vi "Get XNET Signal Names.vi"(6 "Add Info?":bool, 7 "Parent Ref in":T1 format="%.0x", 8 "error in":errorcluster, 9 "Tree In":refnum<vi>, 10 "Parent":string, 11 "Frms":refnum<k21>[](array[refnum])) -> (0 "error out":errorcluster, 1 "Tree Out":refnum<vi>, 3 "XNET Signal Names":refnum<k21>[](array[refnum]))   [LabVIEW 2023, in "J1939 Addon System Explorer.lvlib"]
uses:
  J1939 Addon System Explorer.lvlib
  <vilib>/NI VeriStand/Custom Device API/Custom Device Item Ref.ctl
  <vilib>/NI VeriStand/Custom Device API/Custom Device Channel.ctl
  <vilib>/NI VeriStand/Custom Device API/Custom Device Channel Type.ctl
  Addon Shared/Types/SPN Properties.ctl
  Addon Shared/SubVIs/Constants.vi
  <vilib>/NI VeriStand/Custom Device Tools/Custom Device Utility Library/NI VeriStand - Search for Item by Name.vi
  <vilib>/NI VeriStand/Custom Device API/Set Item Property (U32).vi
  <resource>/objmgr/xnet.rc
  <vilib>/NI VeriStand/Custom Device API/Custom Device API.lvlib
  Addon Shared/J1939 Addon Shared.lvlib
  <vilib>/NI VeriStand/Custom Device Tools/Custom Device Utility Library/Custom Device Utility Library.lvlib
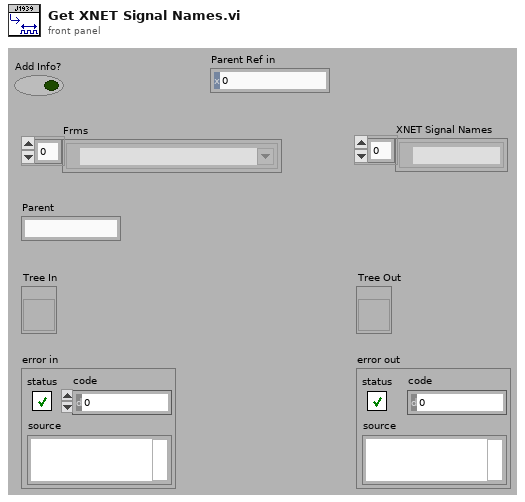
[diagram p1: front panel]
types:
  T1 = typedef "Custom Device API.lvlib/Custom Device Item Ref.ctl" = u64
  T2 = typedef "Custom Device API.lvlib/Custom Device Channel.ctl" = cluster{"Type":T3, "Units":string, "Default Value":dbl, "Faultable":bool, "Scalable":bool}
  T3 = typedef "Custom Device API.lvlib/Custom Device Channel Type.ctl" = enum16{"Input", "Output"}
  T4 = typedef "J1939 Addon Shared.lvlib/SPN Properties.ctl" = cluster{"Bytes":u32, "ScaleFac":dbl, "ScaleOff":dbl}
  T5 = typedef "Custom Device API.lvlib/Custom Device Item Info.ctl" = cluster{"Name":string, "Is Channel":bool, "GUID":string, "Is Waveform":bool}
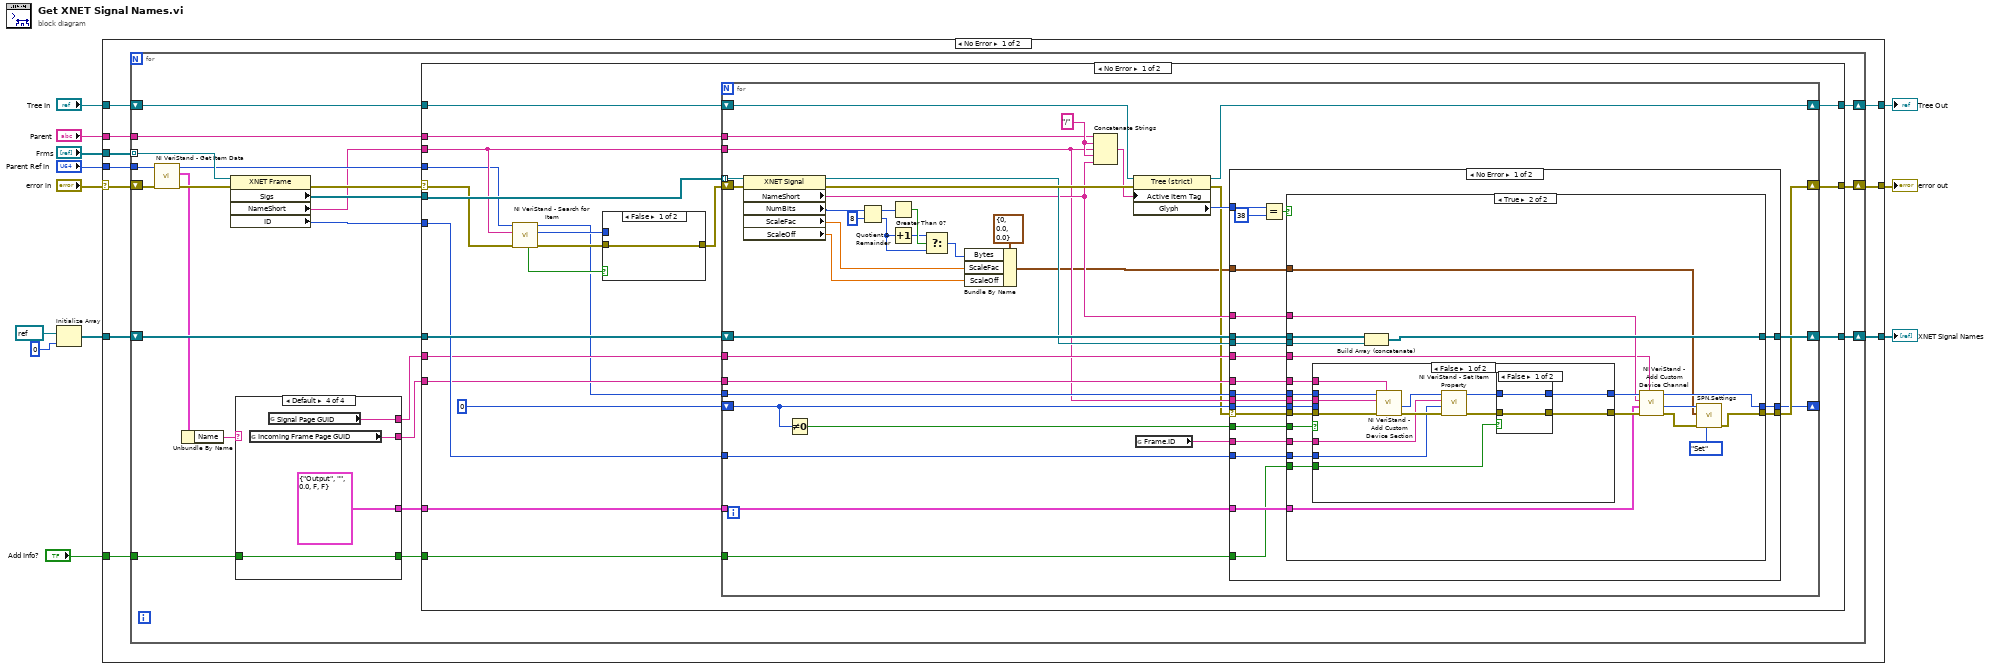
[diagram p0: block diagram]
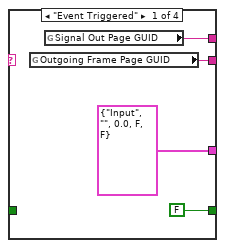
[diagram p2: hidden frame]
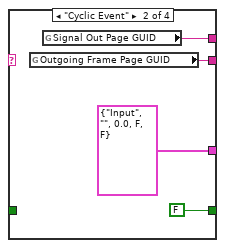
[diagram p3: hidden frame]
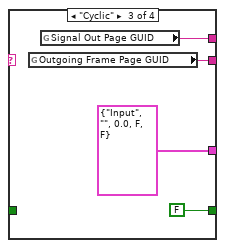
[diagram p4: hidden frame]
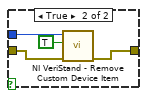
[diagram p5: hidden frame]
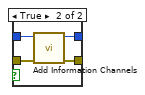
[diagram p7: hidden frame]
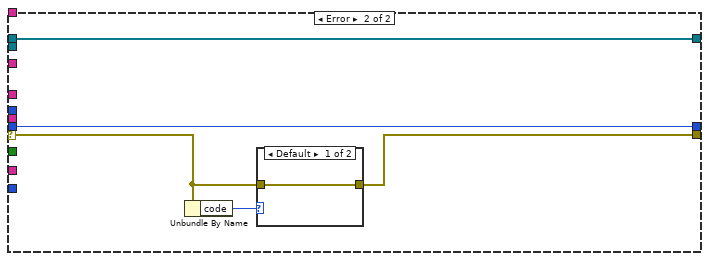
[diagram p9: hidden frame]
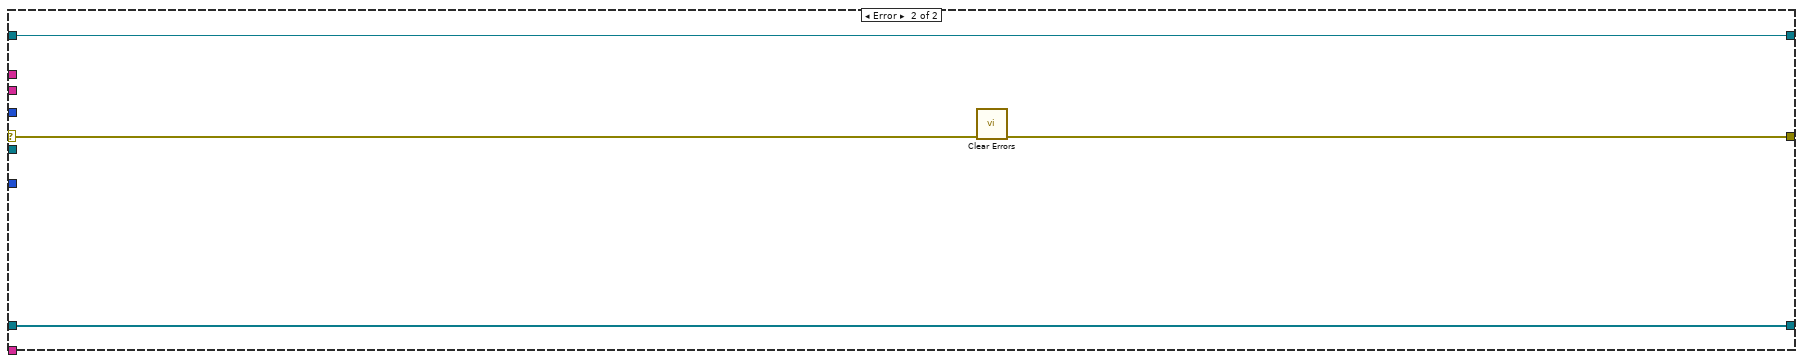
[diagram p11: hidden frame]
diagram:
  n1 = Initialize Array(refnum<k21> refnum ("XNET Signal"), 0 ("dimension size")) -> (w6:refnum<k21>[])
  n2 = case shown="No Error" "error in" {
    selector: "error in" -> [w19 w203]
    tunnel: "Parent" -> [w22 _]
    tunnel: [w21 w203] -> w11
    tunnel: "Frms" -> [w20 _]
    tunnel: [w18 _] -> w8
    tunnel: w6 -> [w17 _]
    tunnel: "Tree In" -> [w16 w202]
    tunnel: [w15 w202] -> w3
    tunnel: "Parent Ref in" -> [w14 _]
    tunnel: "Add Info?" -> [w13 _]
    frame No Error {
      n3 = for {
        shift-right: [w41] -> w21
        shift-left: w19 -> [w35]
        tunnel: w20 -> [w44] mode=indexing
        tunnel: w22 -> [w42]
        shift-right: [w38] -> w18
        shift-left: w17 -> [w39]
        shift-right: [w37] -> w15
        shift-left: w16 -> [w40]
        tunnel: w14 -> [w33]
        tunnel: w13 -> [w26]
        n4 = call <vilib>:"NI VeriStand - Get Item Data.vi"("error in (no error)"=w35, "Item Ref in"=w33) -> ("error out"=w34:errorcluster, "Item Info"=w31:T5, "Item Ref out"=w32:T1)  [unwired: 7 out]
        n5 = Unbundle By Name(w31) -> ("Name"=w30:string)
        n6 = property class="XNET Frame"(reference=w44, error in=w34) -> (error out=w36:errorcluster, "Sigs"=w43:refnum<k21>[], "NameShort"=w28:string, "ID"=w27:u32)  [unwired: 1 out]
        n7 = case shown="Default" w30 {
          tunnel: [T2 {"Type"=enum."Input", "Units"="", "Default Value"=0.0, "Faultable"=FALSE, "Scalable"=FALSE} ("Channel") T2 {"Type"=enum."Input", "Units"="", "Default Value"=0.0, "Faultable"=FALSE, "Scalable"=FALSE} ("Channel") T2 {"Type"=enum."Input", "Units"="", "Default Value"=0.0, "Faultable"=FALSE, "Scalable"=FALSE} ("Channel") T2 {"Type"=enum."Output", "Units"="", "Default Value"=0.0, "Faultable"=FALSE, "Scalable"=FALSE} ("Channel")] -> w29
          tunnel: [FALSE ("Add Info?") FALSE ("Add Info?") FALSE ("Add Info?") w59] -> w25
          tunnel: w26 -> [_ _ _ w59]
          tunnel: [w46 w50 w54 w58] -> w24
          tunnel: [w45 w49 w53 w57] -> w23
          frame "Event Triggered" {
            n8 = global read "Constants.vi" "Outgoing Frame Page GUID"() -> (w46:string)
            n9 = global read "Constants.vi" "Signal Out Page GUID"() -> (w45:string)
          }
          frame "Cyclic Event" {
            n10 = global read "Constants.vi" "Outgoing Frame Page GUID"() -> (w50:string)
            n11 = global read "Constants.vi" "Signal Out Page GUID"() -> (w49:string)
          }
          frame "Cyclic" {
            n12 = global read "Constants.vi" "Outgoing Frame Page GUID"() -> (w54:string)
            n13 = global read "Constants.vi" "Signal Out Page GUID"() -> (w53:string)
          }
          frame Default {
            n14 = global read "Constants.vi" "Incoming Frame Page GUID"() -> (w58:string)
            n15 = global read "Constants.vi" "Signal Page GUID"() -> (w57:string)
          }
        }
        n16 = case shown="No Error" w36 {
          selector: w36 -> [w65 w198]
          tunnel: w43 -> [w81 _]
          tunnel: w28 -> [w63 _]
          tunnel: w42 -> [w80 _]
          tunnel: [w79 w199] -> w41
          tunnel: w40 -> [w78 w200]
          tunnel: w39 -> [w77 w201]
          tunnel: [w76 w201] -> w38
          tunnel: [w75 w200] -> w37
          tunnel: w32 -> [w61 _]
          tunnel: w27 -> [w73 _]
          tunnel: w23 -> [w72 _]
          tunnel: w24 -> [w71 _]
          tunnel: w29 -> [w70 _]
          tunnel: w25 -> [w69 _]
          frame No Error {
            n17 = call-poly <vilib>:"NI VeriStand - Search for Item.vi"("error in"=w65, "Item Name"=w63, "Section Ref in"=w61) -> ("error out"=w66:errorcluster, "Item Ref"=w67:T1, "Section Ref out"=w62:T1, "Found"=w68:bool)  [unwired: 5 in]
            n18 = case shown="False" w68 {
              tunnel: w67 -> [_ w86]
              tunnel: w66 -> [w82 w85]
              tunnel: [w82 w84] -> w64
              frame False {
              }
              frame True {
                n19 = call <vilib>:"NI VeriStand - Remove Custom Device Item.vi"("error in (no error)"=w85, "Force Delete (F)"=TRUE, "Item Ref in"=w86) -> ("error out"=w84:errorcluster)  [unwired: 7 in, 1 out]
              }
            }
            n20 = for {
              tunnel: w81 -> [w123] mode=indexing
              tunnel: w63 -> [w100]
              tunnel: w80 -> [w120]
              shift-right: [w111] -> w79
              shift-left: w64 -> [w122]
              shift-right: [w115] -> w76
              shift-left: w77 -> [w114]
              shift-right: [w112] -> w75
              shift-left: w78 -> [w118]
              tunnel: w62 -> [w110]
              shift-right: [w109] -> _
              shift-left: T1 0 ("Parent Ref out") -> [w108]
              tunnel: w73 -> [w105]
              tunnel: w72 -> [w103]
              tunnel: w71 -> [w102]
              tunnel: w70 -> [w101]
              tunnel: w69 -> [w88]
              w121 = "/" ("string")
              n21 = property class="XNET Signal"(reference=w123, error in=w122) -> (reference out=w113:refnum<k21>, error out=w119:errorcluster, "NameShort"=w106:string, "NumBits"=w99:u32, "ScaleFac"=w92:dbl, "ScaleOff"=w91:dbl)
              n22 = Not Equal To 0?(x=w108) -> (x != 0?=w107:bool)
              n23 = Quotient & Remainder(x=w99, y=u32 8) -> (x-y*floor(x/y)=w97:u32, floor(x/y)=w95:u32)
              n24 = Greater Than 0?(x=w97) -> (x > 0?=w96:bool)
              n25 = Increment(x=w95) -> (x+1=w94:u32)
              n26 = Select(t=w94, s=w96, f=w95) -> (s? t:f=w93:u32)
              n27 = Bundle By Name(cluster=T4 {"Bytes"=0, "ScaleFac"=0.0, "ScaleOff"=0.0}, "Bytes"=w93, "ScaleFac"=w92, "ScaleOff"=w91) -> (w87:T4)
              n28 = Concatenate Strings(w120, w121, w100, w121, w106) -> (w117:string)
              n29 = property class="Tree (strict)"(reference=w118, error in=w119, "Active Item Tag"=w117) -> (reference out=w112:refnum<vi>, error out=w89:errorcluster, "Glyph"=w116:i32)
              n30 = global read "Constants.vi" "Frame.ID"() -> (w104:string)
              n31 = case shown="No Error" w89 {
                selector: w89 -> [w125 w193]
                tunnel: w116 -> [w144 _]
                tunnel: [w141 w195] -> w115
                tunnel: w114 -> [w140 w195]
                tunnel: w113 -> [w139 _]
                tunnel: [w138 w192] -> w111
                tunnel: w110 -> [w137 _]
                tunnel: [w136 w196] -> w109
                tunnel: w108 -> [w135 w196]
                tunnel: w107 -> [w134 _]
                tunnel: w106 -> [w133 _]
                tunnel: w105 -> [w132 _]
                tunnel: w104 -> [w131 _]
                tunnel: w103 -> [w130 _]
                tunnel: w102 -> [w129 _]
                tunnel: w101 -> [w128 _]
                tunnel: w100 -> [w127 _]
                tunnel: w87 -> [w126 _]
                tunnel: w88 -> [w124 _]
                frame No Error {
                  n32 = Equal?(x=w144, y=38) -> (x = y?=w142:bool)
                  n33 = case shown="True" w142 {
                    tunnel: [w147 w168] -> w141
                    tunnel: w140 -> [w147 w170]
                    tunnel: w139 -> [_ w169]
                    tunnel: w134 -> [_ w167]
                    tunnel: w127 -> [_ w166]
                    tunnel: w125 -> [w146 w165]
                    tunnel: [w146 w150] -> w138
                    tunnel: w137 -> [_ w164]
                    tunnel: [w145 w161] -> w136
                    tunnel: w135 -> [w145 w163]
                    tunnel: w133 -> [_ w159]
                    tunnel: w129 -> [_ w158]
                    tunnel: w130 -> [_ w157]
                    tunnel: w132 -> [_ w156]
                    tunnel: w131 -> [_ w155]
                    tunnel: w128 -> [_ w154]
                    tunnel: w126 -> [_ w148]
                    tunnel: w124 -> [_ w153]
                    frame False {
                    }
                    frame True {
                      n34 = case shown="False" w167 {
                        tunnel: w166 -> [w183 _]
                        tunnel: w165 -> [w182 w191]
                        tunnel: [w177 w191] -> w162
                        tunnel: w164 -> [w181 _]
                        tunnel: [w176 w190] -> w160
                        tunnel: w163 -> [_ w190]
                        tunnel: w158 -> [w180 _]
                        tunnel: w156 -> [w171 _]
                        tunnel: w155 -> [w172 _]
                        tunnel: w153 -> [w178 _]
                        frame False {
                          n35 = call <vilib>:"NI VeriStand - Add Custom Device Section.vi"("GUID (Default Section)"=w180, "error in (no error)"=w182, "Section Name"=w183, "Parent Ref in"=w181) -> ("error out"=w174:errorcluster, "Section Ptr"=w179:T1)  [unwired: 4 in, 2 out]
                          n36 = call-poly <vilib>:"NI VeriStand - Set Item Property.vi"("error in (no error)"=w174, "Value"=w171, "Property Name"=w172, "Item Ref in"=w179) -> ("error out"=w173:errorcluster, "Item Ref out"=w175:T1)  [unwired: 5 in, 1 out]
                          n37 = case shown="False" w178 {
                            tunnel: w175 -> [w184 w189]
                            tunnel: [w184 w188] -> w176
                            tunnel: w173 -> [w185 w187]
                            tunnel: [w185 w186] -> w177
                            frame False {
                            }
                            frame True {
                              n38 = call "Add Information Channels.vi"("error in (no error)"=w187, "Node Ptr"=w189) -> ("error out"=w186:errorcluster, "Parent Ref out"=w188:T1)  [unwired: 8 in]
                            }
                          }
                        }
                        frame True {
                        }
                      }
                      n39 = Build Array (concatenate)(w170, w169) -> (w168:refnum<k21>[])
                      n40 = call <vilib>:"NI VeriStand - Add Custom Device Channel.vi"("GUID (Default Channel)"=w157, "error in (no error)"=w162, "Channel"=w154, "Channel Name"=w159, "Parent Ref in"=w160) -> ("error out"=w151:errorcluster, "Channel Ref"=w152:T1, "Parent Ref out"=w161:T1)  [unwired: 3 in, 1 out]
                      n41 = call "SPN.Settings.vi"("Action"=enum8{"Get", "Set"}."Set", "error in (no error)"=w151, "SPN.Settings"=w148, "Item Ref in"=w152) -> ("error out"=w150:errorcluster)  [unwired: 5 in, 2 out]
                    }
                  }
                }
                frame Error {
                  n42 = Unbundle By Name(w193) -> ("code"=w194:i32)
                  n43 = case shown="Default" w194 {
                    tunnel: [w197 _] -> w192
                    tunnel: w193 -> [w197 _]
                    frame Default {
                    }
                    frame 1136 {
                    }
                  }
                }
              }
            }
          }
          frame Error {
            n44 = call <vilib>:"Clear Errors.vi"("error in (no error)"=w198) -> ("error out"=w199:errorcluster)  [unwired: 5 in, 1 out]
          }
        }
      }
    }
    frame Error {
    }
  }
  "error out" <- w11
  "XNET Signal Names" <- w8
  "Tree Out" <- w3
